vi "SubVI_HInf.vi"(8 "error in (no error)":errorcluster, 11 "Raw EEG In":T2) -> (0 "error out":errorcluster, 3 "Clean EEG Out":T1)   [LabVIEW 2020]
uses:
  <extravilib>/ChannelInstances/Stream-a[.](dbl)/)Channel.ctl
  <extravilib>/ChannelInstances/Stream-a[.,.](dbl)/)Channel.ctl
  <extravilib>/ChannelInstances/Stream-a[.](dbl)/EndpointRead.vi
  <extravilib>/ChannelInstances/Stream-a[.,.](dbl)/Endpoint.vi
  <vilib>/Analysis/7linalg.llb/Create Special Real Matrix.vi
  <vilib>/Analysis/Matrix/Numeric/Multiply/Multiply - RM,R.vi
  Global 1.vi
  <extravilib>/ChannelInstances/Stream-a[.](dbl)/)Channel.vi
  <resource>/ChannelSupport/_ChannelSupport/WaitIfNeeded.vi
  <vilib>/Analysis/baseanly.llb/Real Inverse Matrix.vi
  <vilib>/Analysis/Matrix/Numeric/Power Of X/Power Of X - RM,I.vi
  <vilib>/Analysis/Matrix/Numeric/Multiply/Multiply - RM,RM.vi
  <vilib>/Analysis/Matrix/Numeric/Multiply/Multiply - R,RM.vi
  <vilib>/Analysis/Matrix/Numeric/Subtract/Subtract - RM,RM.vi
  <vilib>/Analysis/Matrix/Numeric/Add/Add (Elementwise) - R,RM.vi
  <vilib>/Analysis/Matrix/Numeric/Subtract/Subtract (Elementwise) - R,RM.vi
  <vilib>/Analysis/Matrix/Numeric/Add/Add - RM,RM.vi
  <vilib>/Analysis/Matrix/Numeric/Conversions/Matrix To Array - RM.vi
  <extravilib>/ChannelInstances/Stream-a[.,.](dbl)/)Channel.vi
  <vilib>/Analysis/Matrix/NI_Matrix.lvlib
  <vilib>/Analysis/NI_AALBase.lvlib
  <vilib>/Analysis/NI_AALPro.lvlib
  <extravilib>/ChannelInstances/Stream-a[.](dbl).lvlib
  <extravilib>/ChannelInstances/Stream-a[.,.](dbl).lvlib
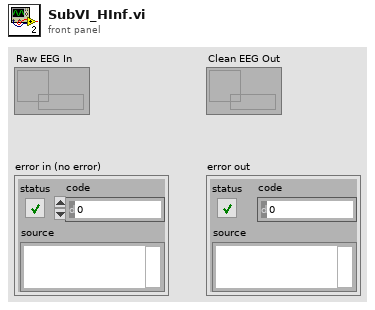
[diagram p1: front panel]
types:
  T1 = typedef "Stream-a[.,.](dbl).lvlib/)Channel.ctl" = refnum<queue>
  T2 = typedef "Stream-a[.](dbl).lvlib/)Channel.ctl" = refnum<queue>
  T3 = typedef "NI_Matrix.lvlib/RealMatrix.ctl" = dbl[][]
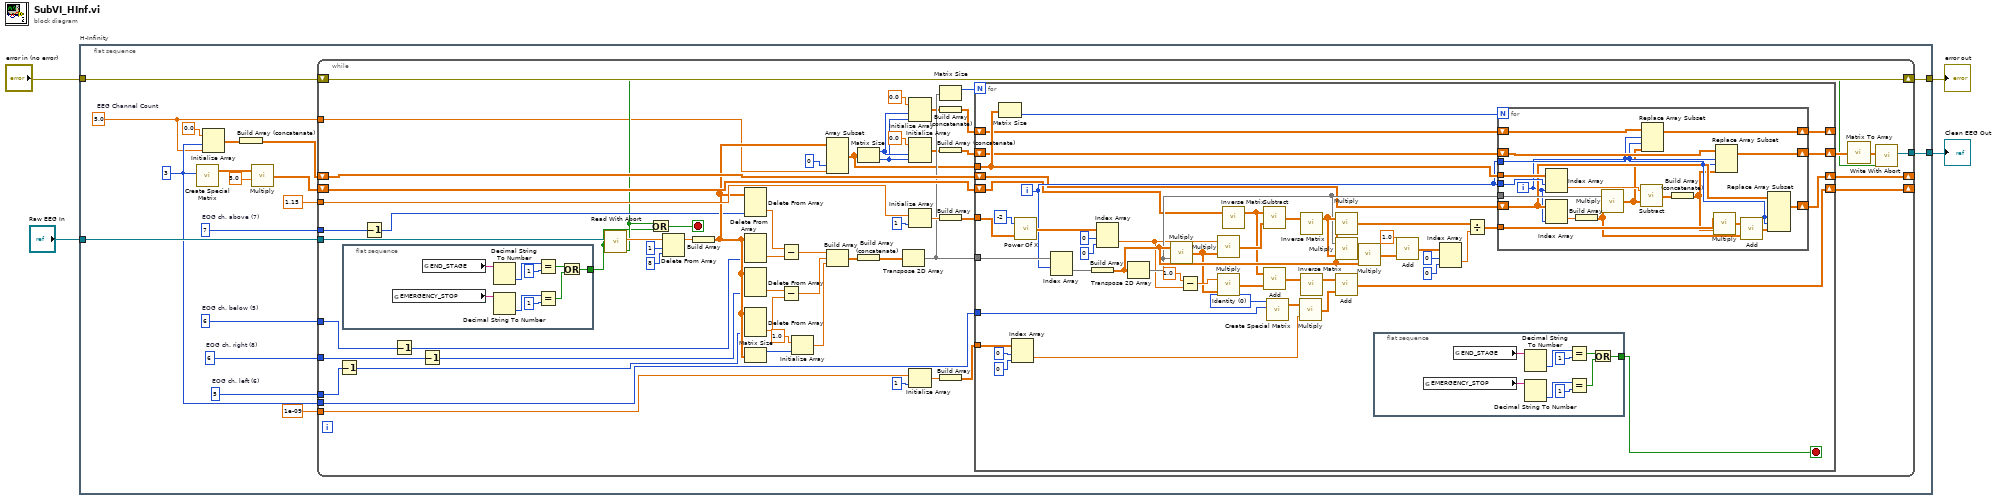
[diagram p0: block diagram]
diagram:
  n1 = flat-sequence "H-Infinity" {
    tunnel: [w22] -> w1
    tunnel: "Raw EEG In" -> [w21]
    tunnel: "error in (no error)" -> [w20]
    tunnel: [w19] -> w2
    frame #0 {
      w5 = 5.0  # EEG Channel Count
      w12 = 3 ("matrix size")
      w11 = 6  # EOG ch. below (5)
      w10 = 7  # EOG ch. above (7)
      w9 = 5  # EOG ch. left (6)
      w8 = 6  # EOG ch. right (8)
      n2 = call-poly <vilib>:"Create Special Matrix.vi"("matrix size"=w12) -> ("Special Matrix"=w17:T3)  [unwired: 4 in, 1 out]
      n3 = Initialize Array(0.0 ("element"), w12, w5) -> (w18:dbl[][])
      n4 = Build Array (concatenate)(w18) -> (w14:T3)
      n5 = call-poly <vilib>:"Multiply.vi"("Real Scalar c"=5.0, "Real Matrix A"=w17) -> ("A * c"=w13:T3)
      n6 = while {
        tunnel: w21 -> [w80]
        tunnel: 1.15 ("gamma (1.15)") -> [w79]
        shift-right: [w78] -> _
        shift-left: w13 -> [w77]
        tunnel: 1e-09 ("q init (1e-10)") -> [w76]
        shift-right: [w74] -> _
        shift-left: w14 -> [w75]
        tunnel: w9 -> [w67]
        tunnel: w10 -> [w66]
        tunnel: w11 -> [w65]
        tunnel: w8 -> [w64]
        shift-right: [w31] -> w22
        shift-left: w20 -> [w31]
        tunnel: [w26] -> w19
        tunnel: w5 -> [w25]
        tunnel: w12 -> [w24]
        stop <- w30 stop-if-true
        n7 = Decrement(x=w67) -> (x-1=w56:i32)
        n8 = flat-sequence {
          tunnel: [w81] -> w23
          frame #0 {
            n9 = global read "Global 1.vi" "EMERGENCY_STOP"() -> (w84:string)
            n10 = global read "Global 1.vi" "END_STAGE"() -> (w89:string)
            n11 = Decimal String To Number(string=w89) -> (number=w88:i32)  [unwired: 2 in, 1 out]
            n12 = Decimal String To Number(string=w84) -> (number=w86:i32)  [unwired: 2 in, 1 out]
            n13 = Equal?(x=w88, y=1) -> (x = y?=w82:bool)
            n14 = Equal?(x=w86, y=1) -> (x = y?=w83:bool)
            n15 = Or(x=w82, y=w83) -> (x .or. y?=w81:bool)
          }
        }
        n16 = Decrement(x=w66) -> (x-1=w53:i32)
        n17 = Decrement(x=w65) -> (x-1=w54:i32)
        n18 = Decrement(x=w64) -> (x-1=w55:i32)
        n19 = call <extravilib>:"Read With Abort.vi"("abort"=w23, "channel"=w80) -> ("element"=w69:dbl[], "aborted?"=w27:bool)  [unwired: 4 in, 4 out]
        n20 = Or(x=w27, y=w23) -> (x .or. y?=w30:bool)
        n21 = Delete From Array(array=w69, length=1, index=8) -> (array with subset deleted=w70:dbl[])  [unwired: 1 out]
        n22 = Build Array(w70) -> (w68:dbl[][])
        n23 = Delete From Array(array=w68, index (col)=w53) -> (deleted portion=w49:dbl[])  [unwired: 2 in, 1 out]
        n24 = Delete From Array(array=w68, index (col)=w54) -> (deleted portion=w52:dbl[])  [unwired: 2 in, 1 out]
        n25 = Delete From Array(array=w68, index (col)=w55) -> (deleted portion=w51:dbl[])  [unwired: 2 in, 1 out]
        n26 = Delete From Array(array=w68, index (col)=w56) -> (deleted portion=w50:dbl[])  [unwired: 2 in, 1 out]
        n27 = Matrix Size(0:w68) -> (1:w41:i32)  [unwired: 1 out]
        n28 = Subtract ("Subtract.vi")(x=w49, y=w52) -> (x-y=w62:dbl[])
        n29 = Subtract ("Subtract.vi")(x=w51, y=w50) -> (x-y=w61:dbl[])
        n30 = Initialize Array(1.0 ("element"), w41) -> (w47:dbl[])
        n31 = Array Subset(array=w68, index (col)=0 ("index"), length (col)=w25) -> (w29:dbl[][])  [unwired: 2 in]
        n32 = Build Array(w62, w61, w47) -> (w34:dbl[][])
        n33 = Matrix Size(0:w29) -> (1:w33:i32, 2:w32:i32)
        n34 = Build Array (concatenate)(w34) -> (w45:T3)
        n35 = Transpose 2D Array(2D array=w45) -> (transposed array=w43:T3)
        n36 = Initialize Array(0.0 ("element"), w33, w32) -> (w39:dbl[][])
        n37 = Initialize Array(0.0 ("element"), w33, w32) -> (w40:dbl[][])
        n38 = Initialize Array(w79, 1 ("dimension size")) -> (w58:dbl[])
        n39 = Initialize Array(w76, 1 ("dimension size")) -> (w59:dbl[])
        n40 = Matrix Size(0:w43) -> (1:w42:i32)  [unwired: 1 out]
        n41 = Build Array (concatenate)(w39) -> (w35:T3)
        n42 = Build Array (concatenate)(w40) -> (w36:T3)
        n43 = Build Array(w58) -> (w44:T3)
        n44 = Build Array(w59) -> (w60:T3)
        n45 = for {
          N: w42 -> [_]
          tunnel: w44 -> [w136]
          tunnel: w43 -> [w134]
          tunnel: w29 -> [w125]
          shift-right: [w104] -> _
          shift-left: w35 -> [w107]
          shift-right: [w105] -> w73
          shift-left: w36 -> [w108]
          shift-right: [w106] -> w74
          shift-left: w75 -> [w109]
          shift-right: [w99] -> w78
          shift-left: w77 -> [w100]
          tunnel: w60 -> [w96]
          tunnel: w24 -> [w91]
          i -> [w110]
          stop <- w90 stop-if-true
          w93 = 0 items=["Identity", "Diagonal", "Toeplitz", "Vandermonde", "Companion", "Hankel", "Hadamard", "Wilkinson", "Hilbert", "Inverse Hilbert", "Rosser", "Pascal"] ("matrix type")
          n46 = Matrix Size(0:w125) -> (2:w126:i32)  [unwired: 1 out]
          n47 = Index Array(array=w96, index (row)=0, index (col)=0 ("disabled index (col)")) -> (element=w98:dbl)
          n48 = call-poly <vilib>:"Power Of X.vi"("Real Matrix A"=w136, "Power n"=-2) -> ("A^n"=w115:T3)
          n49 = Index Array(array=w134, index (row)=w110) -> (element=w137:dbl[])  [unwired: 1 in]
          n50 = Build Array(w137) -> (w130:T3)
          n51 = Index Array(array=w115, index (row)=0, index (col)=0 ("disabled index (col)")) -> (element=w114:dbl)
          n52 = Transpose 2D Array(2D array=w130) -> (transposed array=w128:T3)
          n53 = call-poly <vilib>:"Multiply.vi"("Real Matrix B"=w128, "Real Matrix A"=w130) -> ("A * B"=w103:T3)
          n54 = Subtract(x=1.0, y=w114) -> (x-y=w112:dbl)
          n55 = call-poly <vilib>:"Multiply.vi"("Real Matrix A"=w103, "Real Scalar c"=w114) -> ("c * A"=w102:T3)
          n56 = call-poly <vilib>:"Multiply.vi"("Real Matrix A"=w103, "Real Scalar c"=w112) -> ("c * A"=w111:T3)
          n57 = call-poly <vilib>:"Inverse Matrix.vi"("Input Matrix"=w100) -> ("Inverse Matrix"=w101:T3)  [unwired: 1 in, 1 out]
          n58 = call-poly <vilib>:"Subtract.vi"("Real Matrix B"=w102, "Real Matrix A"=w101) -> ("A - B"=w138:T3)
          n59 = call-poly <vilib>:"Add.vi"("Real Matrix B"=w111, "Real Matrix A"=w101) -> ("A + B"=w116:T3)
          n60 = call-poly <vilib>:"Create Special Matrix.vi"("matrix type"=w93, "matrix size"=w91) -> ("Special Matrix"=w97:T3)  [unwired: 3 in, 1 out]
          n61 = call-poly <vilib>:"Multiply.vi"("Real Scalar c"=w98, "Real Matrix A"=w97) -> ("A * c"=w92:T3)
          n62 = call-poly <vilib>:"Inverse Matrix.vi"("Input Matrix"=w138) -> ("Inverse Matrix"=w132:T3)  [unwired: 1 in, 1 out]
          n63 = call-poly <vilib>:"Inverse Matrix.vi"("Input Matrix"=w116) -> ("Inverse Matrix"=w117:T3)  [unwired: 1 in, 1 out]
          n64 = call-poly <vilib>:"Multiply.vi"("Real Matrix B"=w130, "Real Matrix A"=w132) -> ("A * B"=w122:T3)
          n65 = call-poly <vilib>:"Multiply.vi"("Real Matrix B"=w132, "Real Matrix A"=w128) -> ("A * B"=w131:T3)
          n66 = call-poly <vilib>:"Add.vi"("Real Matrix B"=w92, "Real Matrix A"=w117) -> ("A + B"=w99:T3)
          n67 = call-poly <vilib>:"Multiply.vi"("Real Matrix B"=w130, "Real Matrix A"=w131) -> ("A * B"=w129:T3)
          n68 = flat-sequence {
            tunnel: [w139] -> w90
            frame #0 {
              n69 = global read "Global 1.vi" "EMERGENCY_STOP"() -> (w142:string)
              n70 = global read "Global 1.vi" "END_STAGE"() -> (w147:string)
              n71 = Decimal String To Number(string=w147) -> (number=w146:i32)  [unwired: 2 in, 1 out]
              n72 = Decimal String To Number(string=w142) -> (number=w144:i32)  [unwired: 2 in, 1 out]
              n73 = Equal?(x=w146, y=1) -> (x = y?=w140:bool)
              n74 = Equal?(x=w144, y=1) -> (x = y?=w141:bool)
              n75 = Or(x=w140, y=w141) -> (x .or. y?=w139:bool)
            }
          }
          n76 = call-poly <vilib>:"Add.vi"("Real Matrix A"=w129, "Real Scalar c"=1.0 ("x")) -> ("c + A"=w119:T3)
          n77 = Index Array(array=w119, index (row)=0, index (col)=0 ("disabled index (col)")) -> (element=w118:dbl)
          n78 = Divide(x=w122, y=w118) -> (x/y=w127:T3)
          n79 = for {
            N: w126 -> [_]
            tunnel: w128 -> [w160]
            tunnel: w127 -> [w163]
            tunnel: w110 -> [w164]
            tunnel: w125 -> [w167]
            shift-right: [w161] -> w106
            shift-left: w109 -> [w157]
            shift-right: [w149] -> w104
            shift-left: w107 -> [w151]
            tunnel: w110 -> [w155]
            shift-right: [w154] -> w105
            shift-left: w108 -> [w156]
            i -> [w152]
            n80 = Index Array(array=w167, index (row)=w164, index (col)=w152) -> (element=w158:dbl)
            n81 = Index Array(array=w157, index (col)=w152) -> (element=w165:dbl[])  [unwired: 1 in]
            n82 = Build Array(w165) -> (w159:T3)
            n83 = call-poly <vilib>:"Multiply.vi"("Real Matrix B"=w159, "Real Matrix A"=w160) -> ("A * B"=w150:T3)
            n84 = call-poly <vilib>:"Subtract.vi"("Real Matrix A"=w150, "Real Scalar c"=w158) -> ("c - A"=w166:T3)
            n85 = Replace Array Subset(array=w151, new element=w150, index (row)=w155, index (col)=w152) -> (w149:T3)
            n86 = Build Array (concatenate)(w166) -> (w148:T3)
            n87 = call-poly <vilib>:"Multiply.vi"("Real Matrix B"=w148, "Real Matrix A"=w163) -> ("A * B"=w162:T3)
            n88 = Replace Array Subset(array=w156, new element=w148, index (row)=w155, index (col)=w152) -> (w154:T3)
            n89 = call-poly <vilib>:"Add.vi"("Real Matrix B"=w159, "Real Matrix A"=w162) -> ("A + B"=w153:T3)
            n90 = Replace Array Subset(array=w157, new element=w153, index (dim 2)=w152, index (dim 3)=w152) -> (w161:T3)  [unwired: 2 in]
          }
        }
        n91 = call-poly <vilib>:"Matrix To Array.vi"("Real Matrix"=w73) -> ("Real 2D Array"=w28:dbl[][])
        n92 = call <extravilib>:"Write With Abort.vi"("abort"=w27, "element"=w28) -> ("channel"=w26:T1)  [unwired: 6 in, 3 out]
      }
    }
  }
  "Clean EEG Out" <- w2
  "error out" <- w1
